vi "16T_Merge_Cluster.vi"(1 "16 T Control":T2={"Clamp"=FALSE, "Switch Heater"=FALSE, "Go to Zero"=FALSE, "Go to Set"=FALSE, "Go to Hold"=FALSE, "Setpoint (T)"=3.4572, "Rate (T/min)"=0.0, "Set Rate"=FALSE} {"Rate (T/min)" format="%6_5f"; "Setpoint (T)" format="%#4_5f"}, 2 "16 T Status":T3={"Clamped"=FALSE, "Quenched"=FALSE, "Rate limit"=FALSE, "Persistent"=FALSE, "Hold"=FALSE, "Set"=FALSE, "Zero"=FALSE, "Magnet (T)"=0.0, "Leads (T)"=0.0, "Magnet T (K)"=3.4572, "Switch"=FALSE, "Sweeping"=FALSE} {"Magnet T (K)" format="%#4_5f"; "Leads (T)" format="%6_5f"}) -> (0 "16 T Magnet control":T1={"Clamp"=FALSE, "Switch Heater"=FALSE, "Go to Zero"=FALSE, "Go to set"=FALSE, "Go to Hold"=FALSE, "Clamped"=FALSE, "Quenched"=FALSE, "Rate limit"=FALSE, "Persistent"=FALSE, "Hold"=FALSE, "Set"=FALSE, "Zero"=FALSE, "Magnet (T)"=0.0, "Leads (T)"=0.0, "Magnet T (K)"=3.4572, "Switch"=FALSE, "Setpoint (T)"=3.4572, "Rate (T/min)"=0.0, "Select"=FALSE, "Sweeping"=FALSE} {"Rate (T/min)" format="%6_5f"; "Setpoint (T)" format="%6_5f"; "Magnet T (K)" format="%#4_5f"; "Leads (T)" format="%6_5f"})   [LabVIEW 2016]
uses:
  S16/16T_Status.ctl
  S16/16T_Control.ctl
  S16/16T-Cluster.ctl
panel:
  # "20 T"
  # "20 T"
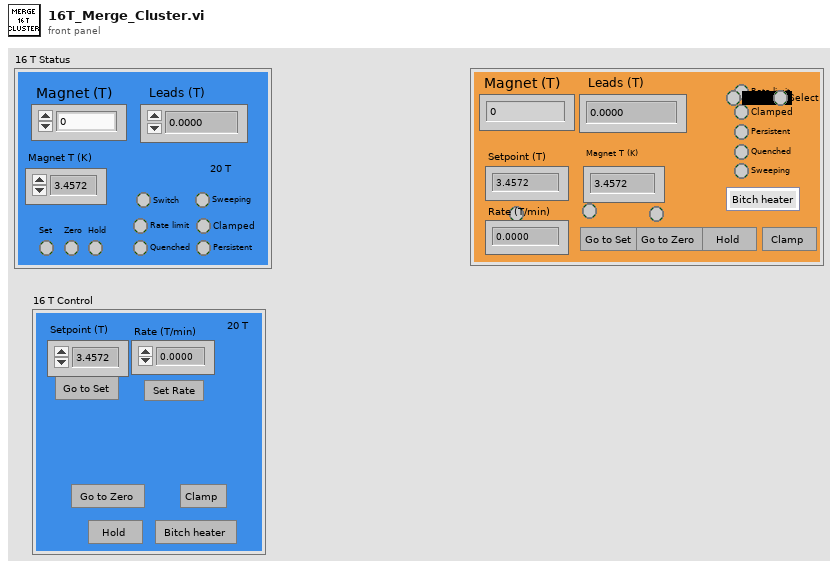
[diagram p1: front panel]
types:
  T1 = typedef "16T-Cluster.ctl" = cluster{"Clamp":bool, "Switch Heater":bool, "Go to Zero":bool, "Go to set":bool, "Go to Hold":bool, "Clamped":bool, "Quenched":bool, "Rate limit":bool, "Persistent":bool, "Hold":bool, "Set":bool, "Zero":bool, "Magnet (T)":dbl, "Leads (T)":dbl, "Magnet T (K)":dbl, "Switch":bool, "Setpoint (T)":dbl, "Rate (T/min)":dbl, "Select":bool, "Sweeping":bool}
  T2 = typedef "16T_Control.ctl" = cluster{"Clamp":bool, "Switch Heater":bool, "Go to Zero":bool, "Go to Set":bool, "Go to Hold":bool, "Setpoint (T)":dbl, "Rate (T/min)":dbl, "Set Rate":bool}
  T3 = typedef "16T_Status.ctl" = cluster{"Clamped":bool, "Quenched":bool, "Rate limit":bool, "Persistent":bool, "Hold":bool, "Set":bool, "Zero":bool, "Magnet (T)":dbl, "Leads (T)":dbl, "Magnet T (K)":dbl, "Switch":bool, "Sweeping":bool}
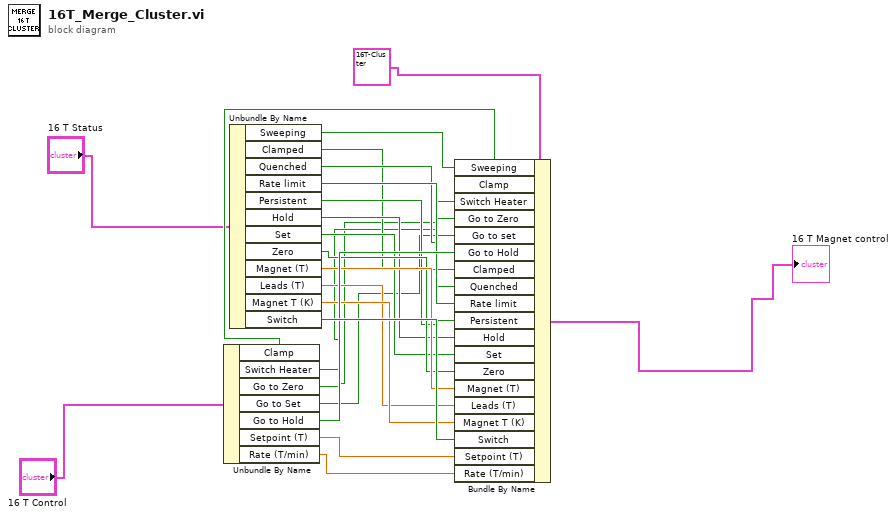
[diagram p0: block diagram]
diagram:
  n1 = Unbundle By Name("16 T Control") -> ("Clamp"=w10:bool, "Switch Heater"=w9:bool, "Go to Zero"=w8:bool, "Go to Set"=w7:bool, "Go to Hold"=w21:bool, "Setpoint (T)"=w23:dbl, "Rate (T/min)"=w6:dbl)
  n2 = Unbundle By Name("16 T Status") -> ("Sweeping"=w1:bool, "Clamped"=w11:bool, "Quenched"=w12:bool, "Rate limit"=w14:bool, "Persistent"=w13:bool, "Hold"=w15:bool, "Set"=w16:bool, "Zero"=w17:bool, "Magnet (T)"=w18:dbl, "Leads (T)"=w19:dbl, "Magnet T (K)"=w20:dbl, "Switch"=w22:bool)
  n3 = Bundle By Name(cluster=T1 {"Clamp"=FALSE, "Switch Heater"=FALSE, "Go to Zero"=FALSE, "Go to set"=FALSE, "Go to Hold"=FALSE, "Clamped"=FALSE, "Quenched"=FALSE, "Rate limit"=FALSE, "Persistent"=FALSE, "Hold"=FALSE, "Set"=FALSE, "Zero"=FALSE, "Magnet (T)"=0.0, "Leads (T)"=0.0, "Magnet T (K)"=3.4572, "Switch"=FALSE, "Setpoint (T)"=3.4572, "Rate (T/min)"=0.0, "Select"=FALSE, "Sweeping"=FALSE} ("16 T Magnet control 2"), "Sweeping"=w1, "Clamp"=w10, "Switch Heater"=w9, "Go to Zero"=w8, "Go to set"=w7, "Go to Hold"=w21, "Clamped"=w11, "Quenched"=w12, "Rate limit"=w14, "Persistent"=w13, "Hold"=w15, "Set"=w16, "Zero"=w17, "Magnet (T)"=w18, "Leads (T)"=w19, "Magnet T (K)"=w20, "Switch"=w22, "Setpoint (T)"=w23, "Rate (T/min)"=w6) -> (→"16 T Magnet control":T1)
